vi "glueing_proc_switch_repTest.vi"() -> ()   [LabVIEW 2015]
panel:
  in  "STOP REP.":bool
  in  "KILL":bool
  in  "PAUSE":bool
  in  "RESUME":bool
  in  "QUIT":bool
  out "output":string
  out "command":string
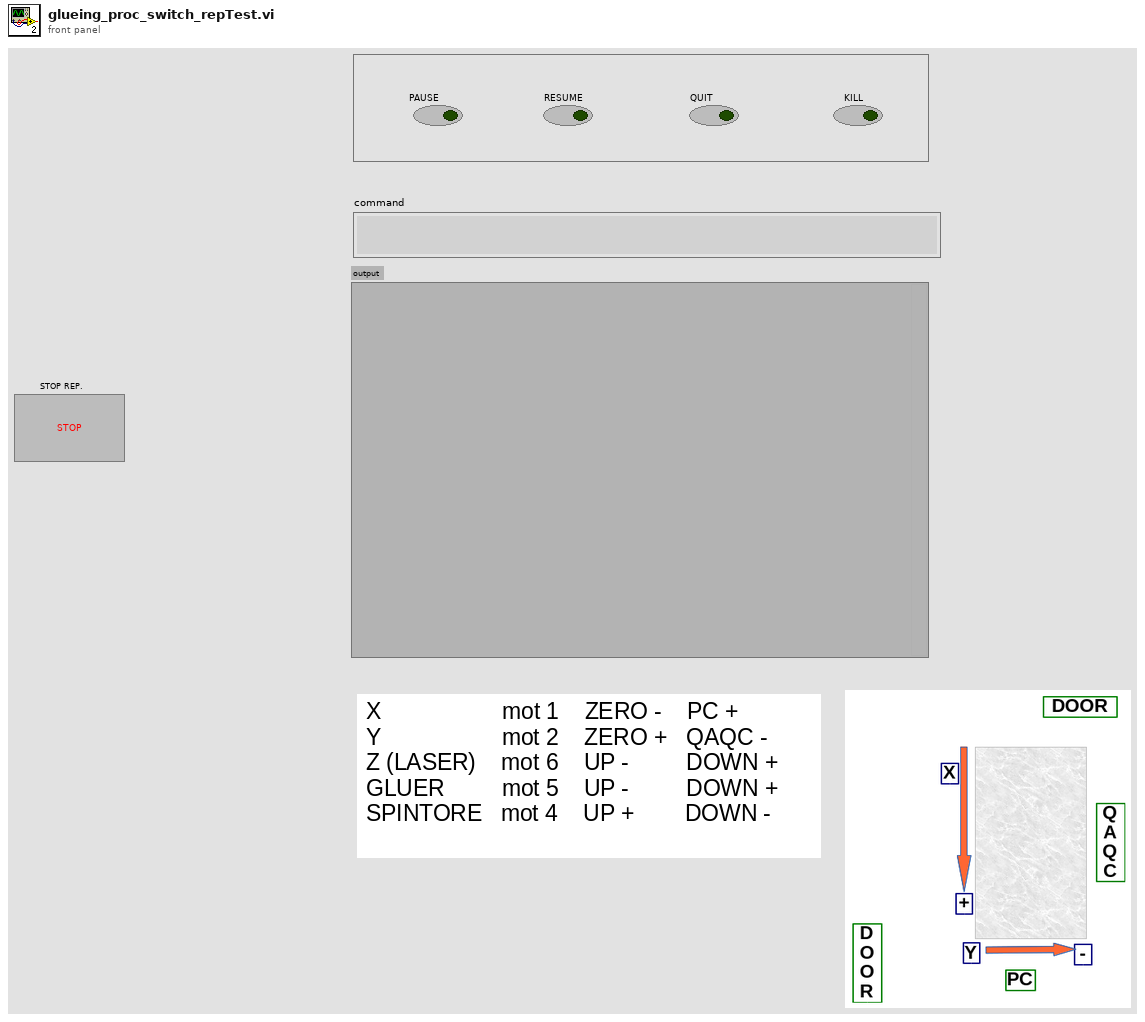
[diagram p1: front panel]
types:
  T1 = enum16{"open", "replace", "create", "open or create", "replace or create", "replace or create with confirmation"}
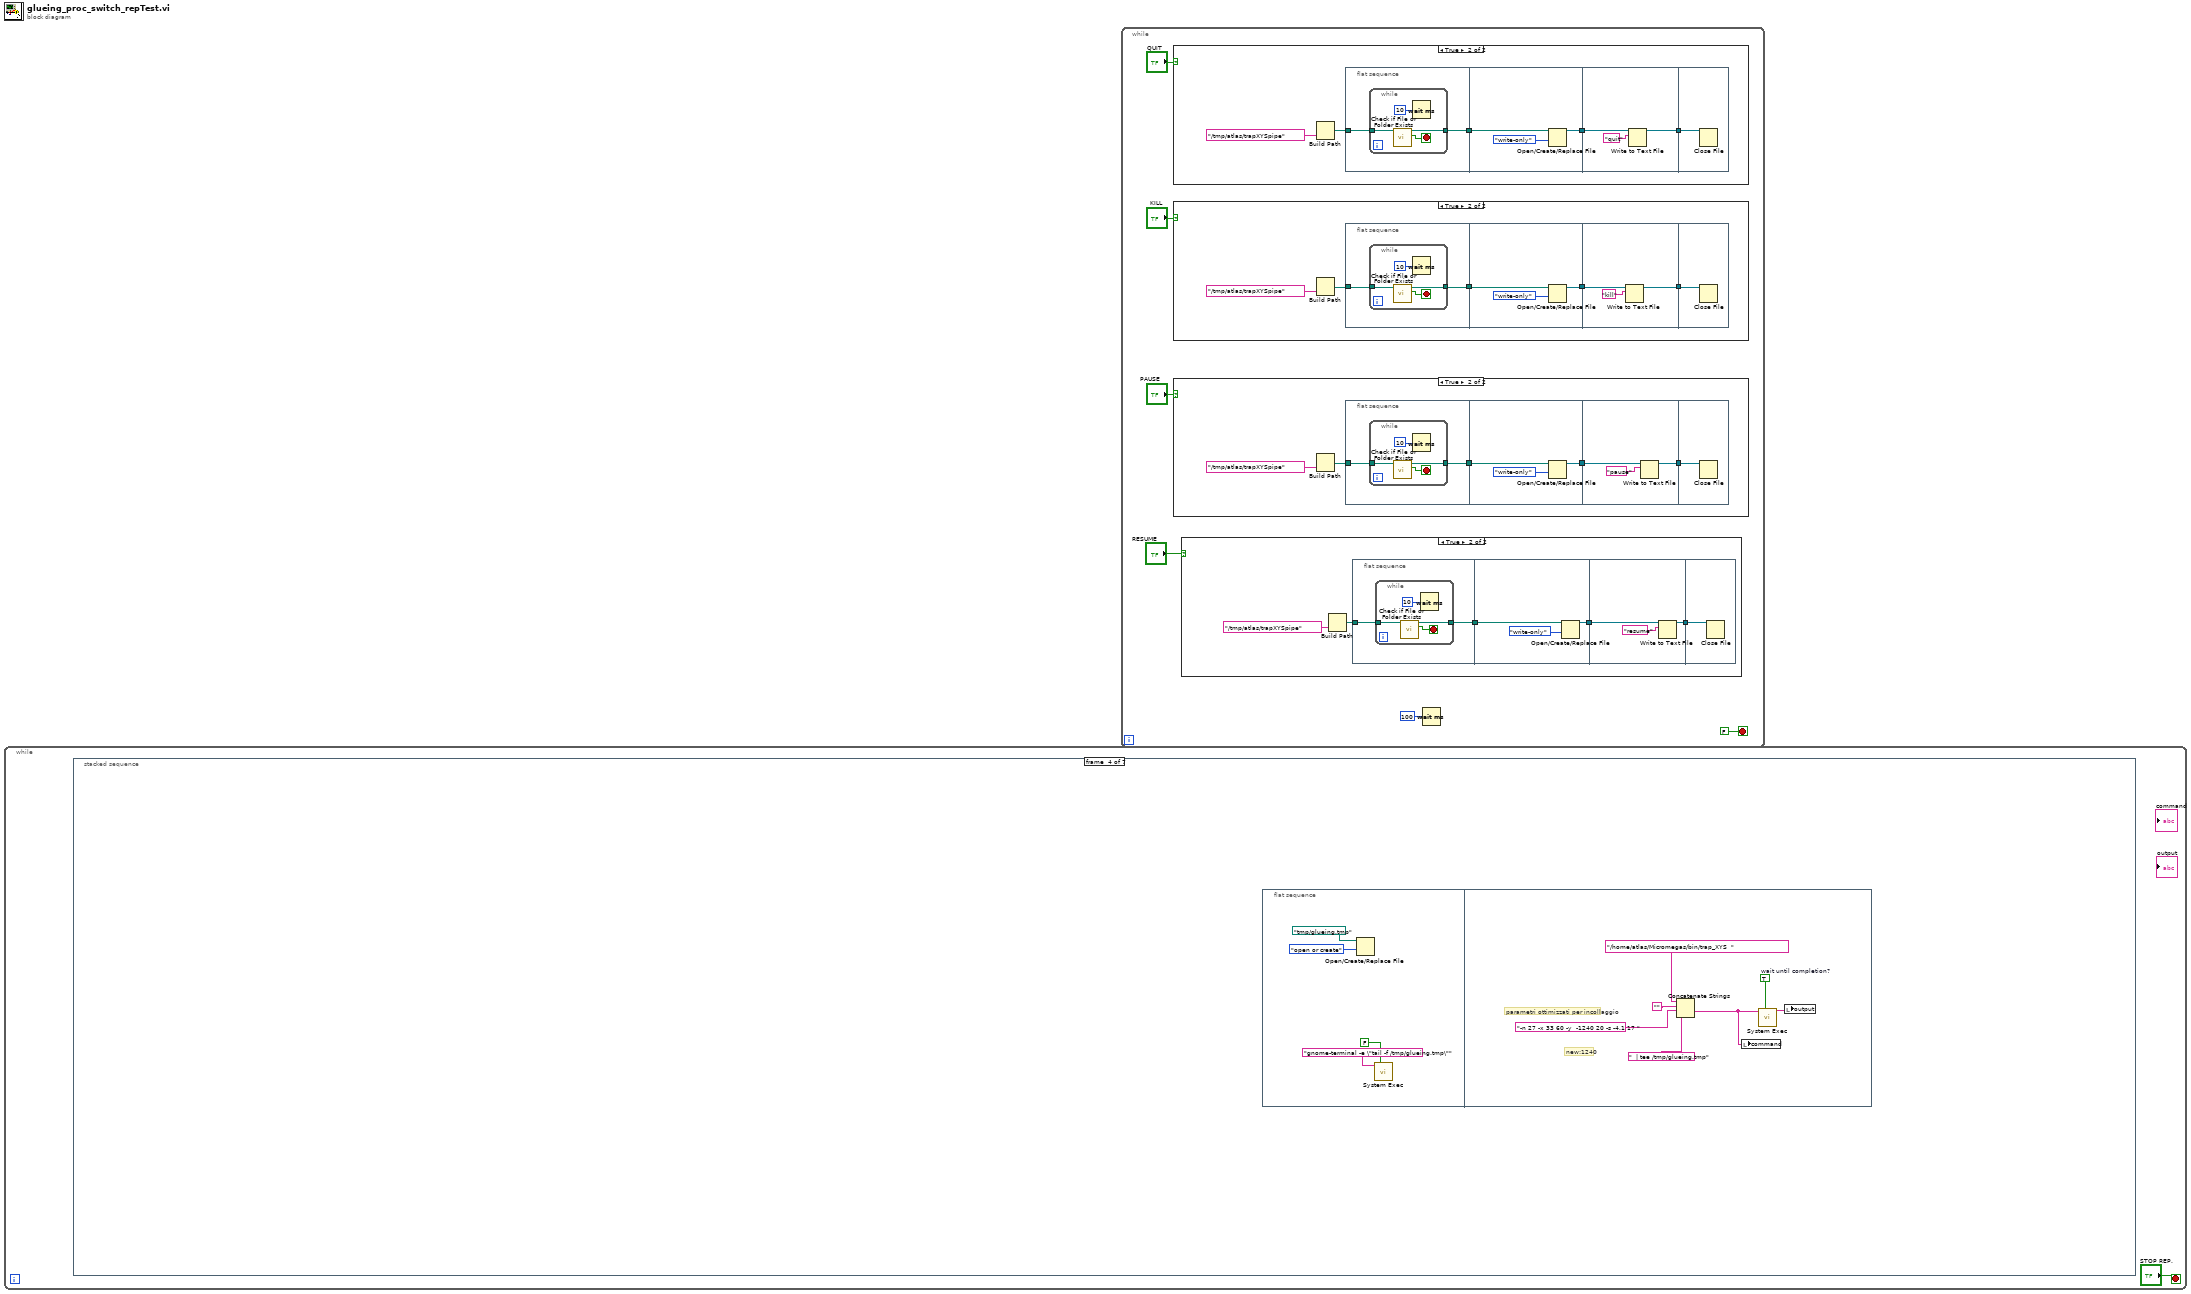
[diagram p0: block diagram]
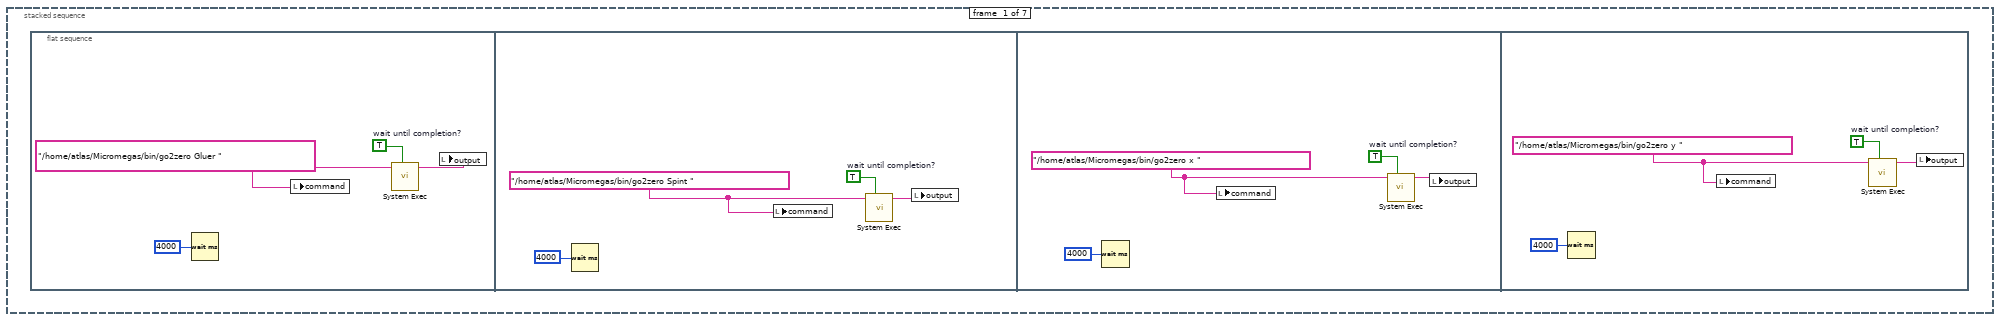
[diagram p2: hidden frame]
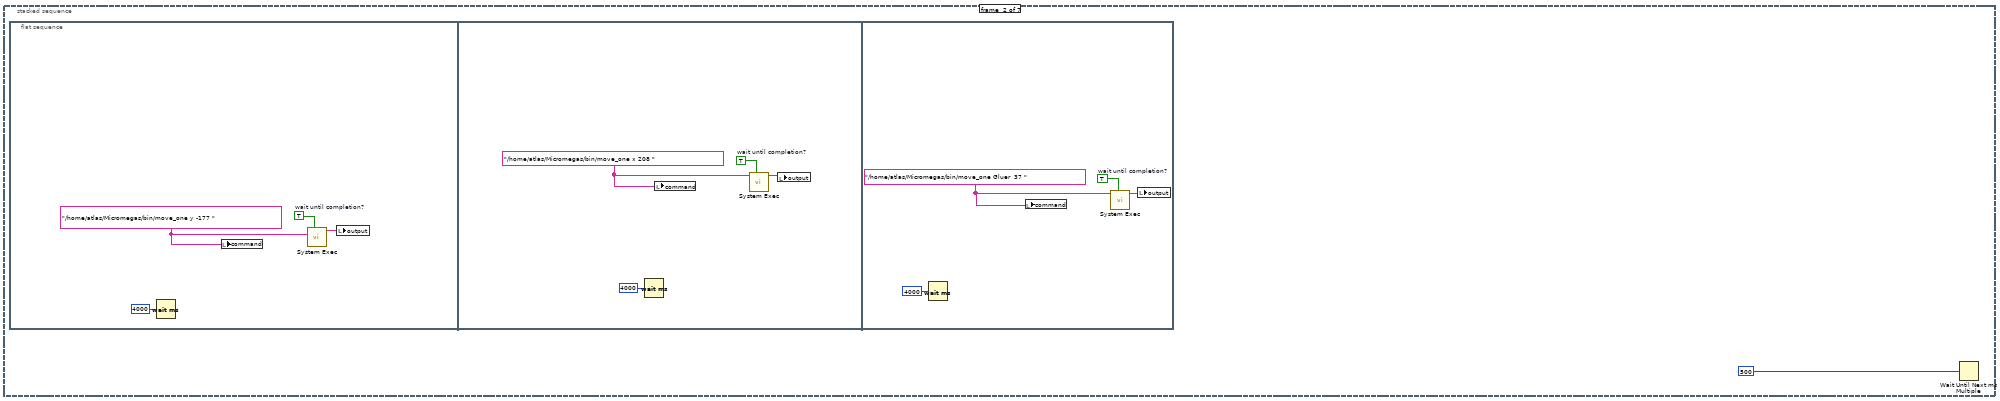
[diagram p3: hidden frame]
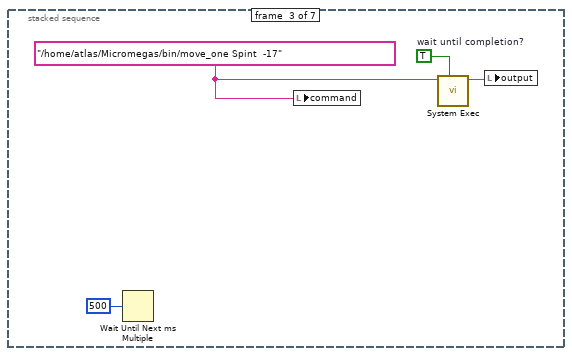
[diagram p4: hidden frame]
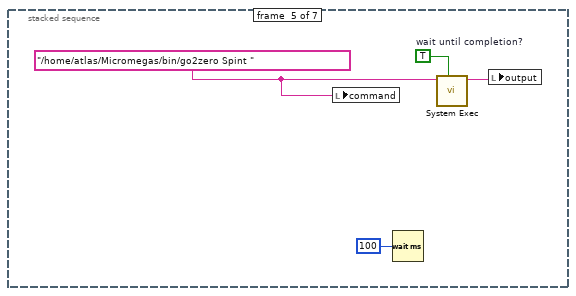
[diagram p5: hidden frame]
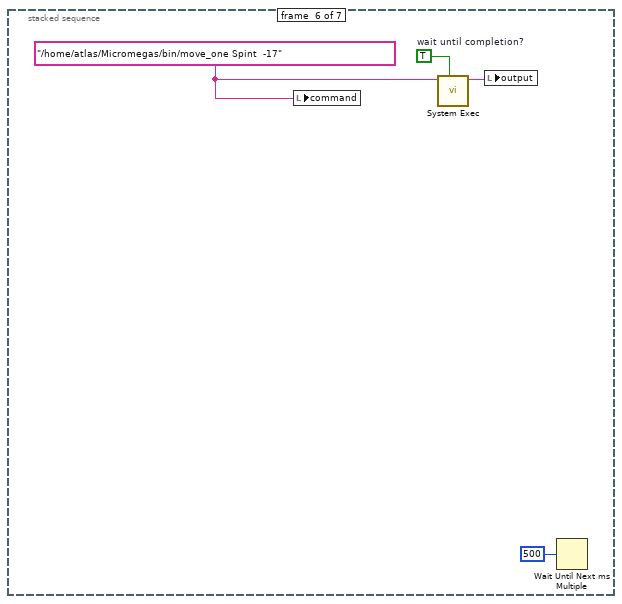
[diagram p6: hidden frame]
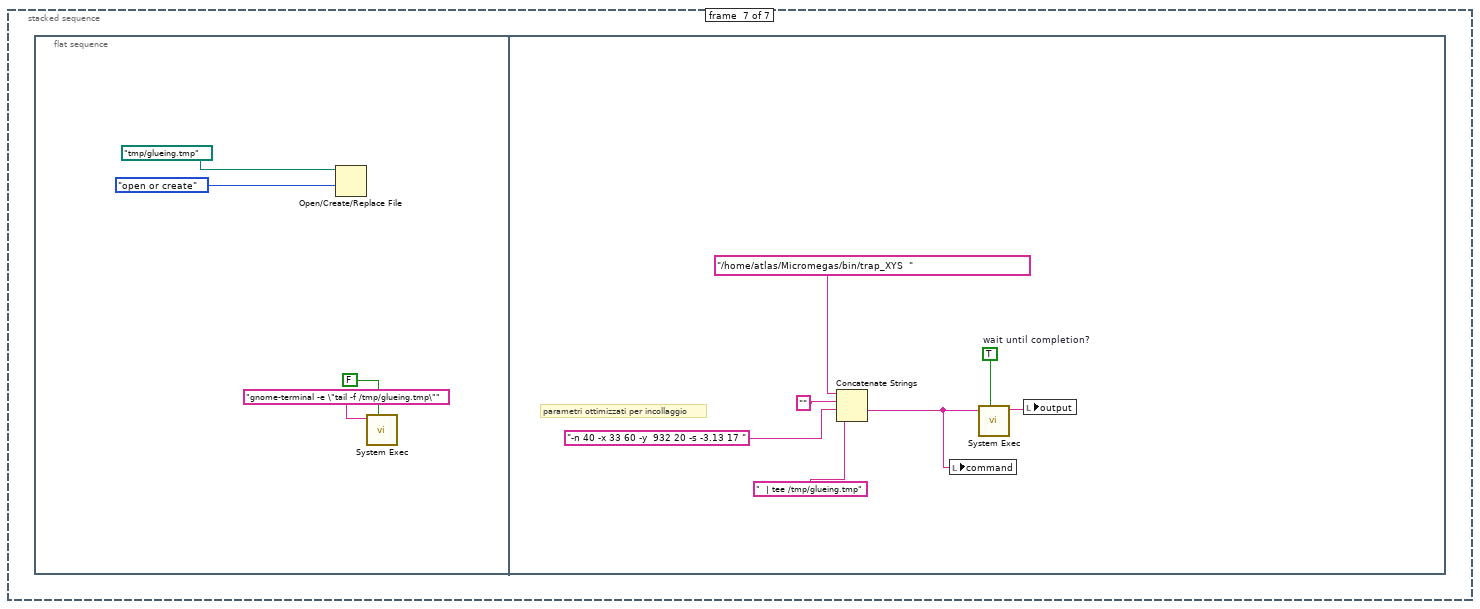
[diagram p7: hidden frame]
diagram:
  n1 = while {
    stop <- "STOP REP." stop-if-true
    n2 = stacked-sequence {
      frame #0 {
        n3 = flat-sequence {
          frame #0 {
            w4 = "/home/atlas/Micromegas/bin/go2zero Gluer " ("string")
            w5 = TRUE  # wait until completion?
            n4 = Wait (ms)(milliseconds to wait=u32 4000) -> ()  [unwired: 1 out]
            n5 = local write "command"(w4) -> ()
            n6 = call <vilib>:"System Exec.vi"("wait until completion? (T)"=w5, "command line"=w4) -> ("standard output"=w3:string)  [unwired: 6 in, 3 out]
            n7 = local write "output"(w3) -> ()
          }
          frame #1 {
            w9 = "/home/atlas/Micromegas/bin/go2zero Spint " ("string")
            w7 = TRUE  # wait until completion?
            n8 = Wait (ms)(milliseconds to wait=u32 4000) -> ()  [unwired: 1 out]
            n9 = local write "command"(w9) -> ()
            n10 = call <vilib>:"System Exec.vi"("wait until completion? (T)"=w7, "command line"=w9) -> ("standard output"=w8:string)  [unwired: 6 in, 3 out]
            n11 = local write "output"(w8) -> ()
          }
          frame #2 {
            w12 = "/home/atlas/Micromegas/bin/go2zero x " ("string")
            w11 = TRUE  # wait until completion?
            n12 = Wait (ms)(milliseconds to wait=u32 4000) -> ()  [unwired: 1 out]
            n13 = local write "command"(w12) -> ()
            n14 = call <vilib>:"System Exec.vi"("wait until completion? (T)"=w11, "command line"=w12) -> ("standard output"=w13:string)  [unwired: 6 in, 3 out]
            n15 = local write "output"(w13) -> ()
          }
          frame #3 {
            w16 = "/home/atlas/Micromegas/bin/go2zero y " ("string")
            w15 = TRUE  # wait until completion?
            n16 = Wait (ms)(milliseconds to wait=u32 4000) -> ()  [unwired: 1 out]
            n17 = local write "command"(w16) -> ()
            n18 = call <vilib>:"System Exec.vi"("wait until completion? (T)"=w15, "command line"=w16) -> ("standard output"=w17:string)  [unwired: 6 in, 3 out]
            n19 = local write "output"(w17) -> ()
          }
        }
      }
      frame #1 {
        n20 = flat-sequence {
          frame #0 {
            w21 = "/home/atlas/Micromegas/bin/move_one y -177 " ("string")
            w19 = TRUE  # wait until completion?
            n21 = Wait (ms)(milliseconds to wait=u32 4000) -> ()  [unwired: 1 out]
            n22 = local write "command"(w21) -> ()
            n23 = call <vilib>:"System Exec.vi"("wait until completion? (T)"=w19, "command line"=w21) -> ("standard output"=w20:string)  [unwired: 6 in, 3 out]
            n24 = local write "output"(w20) -> ()
          }
          frame #1 {
            w25 = "/home/atlas/Micromegas/bin/move_one x 208 " ("string")
            w23 = TRUE  # wait until completion?
            n25 = Wait (ms)(milliseconds to wait=u32 4000) -> ()  [unwired: 1 out]
            n26 = local write "command"(w25) -> ()
            n27 = call <vilib>:"System Exec.vi"("wait until completion? (T)"=w23, "command line"=w25) -> ("standard output"=w24:string)  [unwired: 6 in, 3 out]
            n28 = local write "output"(w24) -> ()
          }
          frame #2 {
            w30 = "/home/atlas/Micromegas/bin/move_one Gluer  37 " ("string")
            w28 = TRUE  # wait until completion?
            n29 = Wait (ms)(milliseconds to wait=u32 4000) -> ()  [unwired: 1 out]
            n30 = local write "command"(w30) -> ()
            n31 = call <vilib>:"System Exec.vi"("wait until completion? (T)"=w28, "command line"=w30) -> ("standard output"=w29:string)  [unwired: 6 in, 3 out]
            n32 = local write "output"(w29) -> ()
          }
        }
        n33 = Wait Until Next ms Multiple(millisecond multiple=u32 500) -> ()  [unwired: 1 out]
      }
      frame #2 {
        w31 = "/home/atlas/Micromegas/bin/move_one Spint  -17" ("string")
        w33 = TRUE  # wait until completion?
        n34 = Wait Until Next ms Multiple(millisecond multiple=u32 500) -> ()  [unwired: 1 out]
        n35 = local write "command"(w31) -> ()
        n36 = call <vilib>:"System Exec.vi"("wait until completion? (T)"=w33, "command line"=w31) -> ("standard output"=w32:string)  [unwired: 6 in, 3 out]
        n37 = local write "output"(w32) -> ()
      }
      frame #3 {
        n38 = flat-sequence {
          frame #0 {
            n39 = Open/Create/Replace File(file path (use dialog)=path "/tmp/glueing.tmp", operation (0:open)=T1."open or create") -> ()  [unwired: 4 in, 3 out]
            n40 = call <vilib>:"System Exec.vi"("wait until completion? (T)"=FALSE, "command line"="gnome-terminal -e \"tail -f /tmp/glueing.tmp\"" ("logwindow")) -> ()  [unwired: 6 in, 4 out]
          }
          frame #1 {
            w45 = TRUE  # wait until completion?
            # "new:1240"
            # "parametri ottimizzati per incollaggio"
            n41 = Concatenate Strings("/home/atlas/Micromegas/bin/trap_XYS  " ("string"), "" ("string"), "-n 27 -x 33 60 -y  -1240 20 -s -4.1 17 " ("string"), "  | tee /tmp/glueing.tmp" ("string")) -> (w40:string)
            n42 = local write "command"(w40) -> ()
            n43 = call <vilib>:"System Exec.vi"("wait until completion? (T)"=w45, "command line"=w40) -> ("standard output"=w39:string)  [unwired: 6 in, 3 out]
            n44 = local write "output"(w39) -> ()
          }
        }
      }
      frame #4 {
        w46 = "/home/atlas/Micromegas/bin/go2zero Spint " ("string")
        w48 = TRUE  # wait until completion?
        n45 = local write "command"(w46) -> ()
        n46 = Wait (ms)(milliseconds to wait=u32 100) -> ()  [unwired: 1 out]
        n47 = call <vilib>:"System Exec.vi"("wait until completion? (T)"=w48, "command line"=w46) -> ("standard output"=w47:string)  [unwired: 6 in, 3 out]
        n48 = local write "output"(w47) -> ()
      }
      frame #5 {
        w50 = "/home/atlas/Micromegas/bin/move_one Spint  -17" ("string")
        w52 = TRUE  # wait until completion?
        n49 = local write "command"(w50) -> ()
        n50 = call <vilib>:"System Exec.vi"("wait until completion? (T)"=w52, "command line"=w50) -> ("standard output"=w51:string)  [unwired: 6 in, 3 out]
        n51 = local write "output"(w51) -> ()
        n52 = Wait Until Next ms Multiple(millisecond multiple=u32 500) -> ()  [unwired: 1 out]
      }
      frame #6 {
        n53 = flat-sequence {
          frame #0 {
            n54 = Open/Create/Replace File(file path (use dialog)=path "/tmp/glueing.tmp", operation (0:open)=T1."open or create") -> ()  [unwired: 4 in, 3 out]
            n55 = call <vilib>:"System Exec.vi"("wait until completion? (T)"=FALSE, "command line"="gnome-terminal -e \"tail -f /tmp/glueing.tmp\"" ("logwindow")) -> ()  [unwired: 6 in, 4 out]
          }
          frame #1 {
            w64 = TRUE  # wait until completion?
            # "parametri ottimizzati per incollaggio"
            n56 = Concatenate Strings("/home/atlas/Micromegas/bin/trap_XYS  " ("string"), "" ("string"), "-n 40 -x 33 60 -y  932 20 -s -3.13 17 " ("string"), "  | tee /tmp/glueing.tmp" ("string")) -> (w59:string)
            n57 = local write "command"(w59) -> ()
            n58 = call <vilib>:"System Exec.vi"("wait until completion? (T)"=w64, "command line"=w59) -> ("standard output"=w58:string)  [unwired: 6 in, 3 out]
            n59 = local write "output"(w58) -> ()
          }
        }
      }
    }
  }
  n60 = while {
    stop <- FALSE stop-if-true
    n61 = case shown="True" "QUIT" {
      frame False {
      }
      frame True {
        n62 = Build Path(name or relative path="/tmp/atlas/trapXYSpipe" ("string")) -> (appended path=w125:path)  [unwired: 1 in]
        n63 = flat-sequence {
          tunnel: [w131] -> w129
          tunnel: w125 -> [w130]
          tunnel: w129 -> [w138]
          tunnel: [w136] -> w128
          tunnel: w128 -> [w141]
          tunnel: [w140] -> w127
          tunnel: w127 -> [w142]
          frame #0 {
            n64 = while {
              tunnel: [w133] -> w131
              tunnel: w130 -> [w132]
              stop <- w134 stop-if-true
              n65 = call <vilib>:"Check if File or Folder Exists.vi"("path"=w132) -> ("file or folder exists?"=w134:bool, "dup path"=w133:path)  [unwired: 8 in, 1 out]
              n66 = Wait (ms)(milliseconds to wait=u32 10) -> ()  [unwired: 1 out]
            }
          }
          frame #1 {
            n67 = Open/Create/Replace File(file path (use dialog)=w138, access (0:read/write)=enum16{"read/write", "read-only", "write-only"}."write-only") -> (refnum out=w136:refnum<file>)  [unwired: 4 in, 2 out]
          }
          frame #2 {
            n68 = Write to Text File(file (use dialog)=w141, text="quit") -> (refnum out=w140:refnum<file>)  [unwired: 2 in, 2 out]
          }
          frame #3 {
            n69 = Close File(refnum=w142) -> ()  [unwired: 1 in, 2 out]
          }
        }
      }
    }
    n70 = case shown="True" "KILL" {
      frame False {
      }
      frame True {
        n71 = Build Path(name or relative path="/tmp/atlas/trapXYSpipe" ("string")) -> (appended path=w89:path)  [unwired: 1 in]
        n72 = flat-sequence {
          tunnel: [w95] -> w93
          tunnel: w89 -> [w94]
          tunnel: w93 -> [w102]
          tunnel: [w100] -> w92
          tunnel: w92 -> [w105]
          tunnel: [w104] -> w91
          tunnel: w91 -> [w106]
          frame #0 {
            n73 = while {
              tunnel: [w97] -> w95
              tunnel: w94 -> [w96]
              stop <- w98 stop-if-true
              n74 = call <vilib>:"Check if File or Folder Exists.vi"("path"=w96) -> ("file or folder exists?"=w98:bool, "dup path"=w97:path)  [unwired: 8 in, 1 out]
              n75 = Wait (ms)(milliseconds to wait=u32 10) -> ()  [unwired: 1 out]
            }
          }
          frame #1 {
            n76 = Open/Create/Replace File(file path (use dialog)=w102, access (0:read/write)=enum16{"read/write", "read-only", "write-only"}."write-only") -> (refnum out=w100:refnum<file>)  [unwired: 4 in, 2 out]
          }
          frame #2 {
            n77 = Write to Text File(file (use dialog)=w105, text="kill") -> (refnum out=w104:refnum<file>)  [unwired: 2 in, 2 out]
          }
          frame #3 {
            n78 = Close File(refnum=w106) -> ()  [unwired: 1 in, 2 out]
          }
        }
      }
    }
    n79 = case shown="True" "PAUSE" {
      frame False {
      }
      frame True {
        n80 = Build Path(name or relative path="/tmp/atlas/trapXYSpipe" ("string")) -> (appended path=w71:path)  [unwired: 1 in]
        n81 = flat-sequence {
          tunnel: [w77] -> w75
          tunnel: w71 -> [w76]
          tunnel: w75 -> [w84]
          tunnel: [w82] -> w74
          tunnel: w74 -> [w87]
          tunnel: [w86] -> w73
          tunnel: w73 -> [w88]
          frame #0 {
            n82 = while {
              tunnel: [w79] -> w77
              tunnel: w76 -> [w78]
              stop <- w80 stop-if-true
              n83 = call <vilib>:"Check if File or Folder Exists.vi"("path"=w78) -> ("file or folder exists?"=w80:bool, "dup path"=w79:path)  [unwired: 8 in, 1 out]
              n84 = Wait (ms)(milliseconds to wait=u32 10) -> ()  [unwired: 1 out]
            }
          }
          frame #1 {
            n85 = Open/Create/Replace File(file path (use dialog)=w84, access (0:read/write)=enum16{"read/write", "read-only", "write-only"}."write-only") -> (refnum out=w82:refnum<file>)  [unwired: 4 in, 2 out]
          }
          frame #2 {
            n86 = Write to Text File(file (use dialog)=w87, text="pause") -> (refnum out=w86:refnum<file>)  [unwired: 2 in, 2 out]
          }
          frame #3 {
            n87 = Close File(refnum=w88) -> ()  [unwired: 1 in, 2 out]
          }
        }
      }
    }
    n88 = case shown="True" "RESUME" {
      frame False {
      }
      frame True {
        n89 = Build Path(name or relative path="/tmp/atlas/trapXYSpipe" ("string")) -> (appended path=w107:path)  [unwired: 1 in]
        n90 = flat-sequence {
          tunnel: [w113] -> w111
          tunnel: w107 -> [w112]
          tunnel: w111 -> [w120]
          tunnel: [w118] -> w110
          tunnel: w110 -> [w123]
          tunnel: [w122] -> w109
          tunnel: w109 -> [w124]
          frame #0 {
            n91 = while {
              tunnel: [w115] -> w113
              tunnel: w112 -> [w114]
              stop <- w116 stop-if-true
              n92 = call <vilib>:"Check if File or Folder Exists.vi"("path"=w114) -> ("file or folder exists?"=w116:bool, "dup path"=w115:path)  [unwired: 8 in, 1 out]
              n93 = Wait (ms)(milliseconds to wait=u32 10) -> ()  [unwired: 1 out]
            }
          }
          frame #1 {
            n94 = Open/Create/Replace File(file path (use dialog)=w120, access (0:read/write)=enum16{"read/write", "read-only", "write-only"}."write-only") -> (refnum out=w118:refnum<file>)  [unwired: 4 in, 2 out]
          }
          frame #2 {
            n95 = Write to Text File(file (use dialog)=w123, text="resume") -> (refnum out=w122:refnum<file>)  [unwired: 2 in, 2 out]
          }
          frame #3 {
            n96 = Close File(refnum=w124) -> ()  [unwired: 1 in, 2 out]
          }
        }
      }
    }
    n97 = Wait (ms)(milliseconds to wait=100) -> ()  [unwired: 1 out]
  }
